vi "Post-Build Custom Action.vi"(10 "Variant":variant) -> (0 "error out":errorcluster)   [LabVIEW 2019]
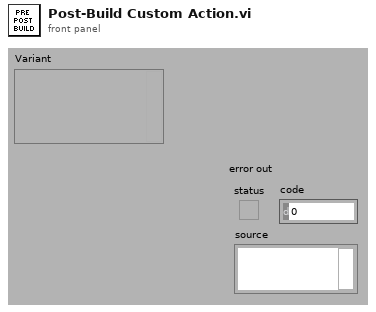
[diagram p1: front panel]
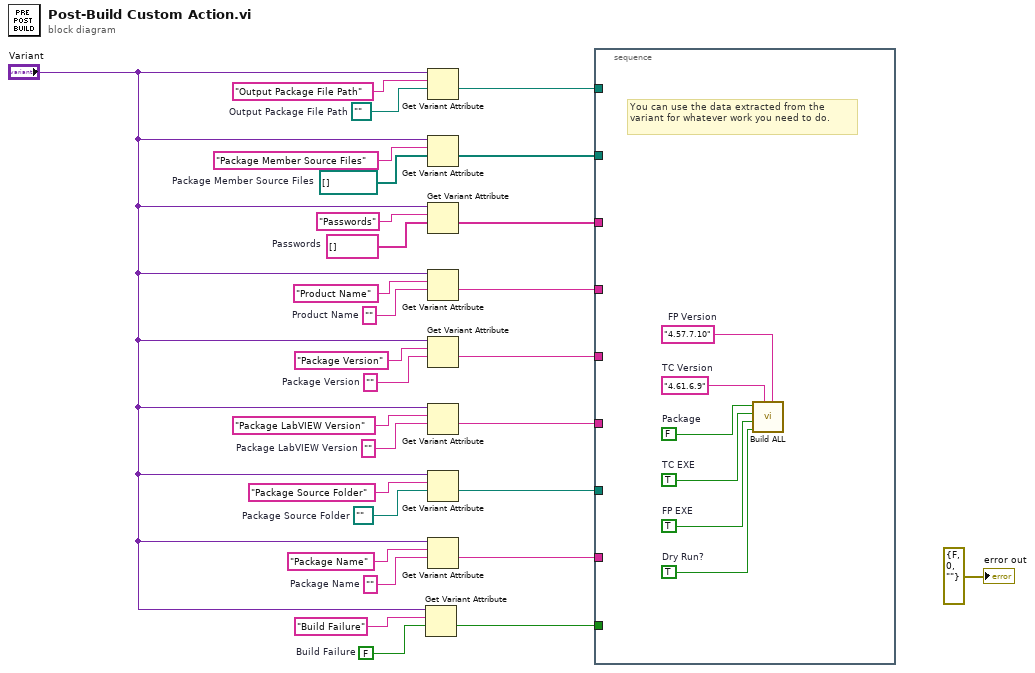
[diagram p0: block diagram]
diagram:
  w3 = FALSE  # Build Failure
  w13 = path ""  # Package Source Folder
  w14 = ""  # Package Name
  w17 = ""  # Package LabVIEW Version
  w19 = ""  # Package Version
  w21 = ""  # Product Name
  w24 = string[] []  # Passwords
  w26 = path[] []  # Package Member Source Files
  w28 = path ""  # Output Package File Path
  n1 = Get Variant Attribute(Variant="Variant", name="Build Failure", default value (empty Variant)=w3) -> (value=w1:bool)  [unwired: 1 in, 3 out]
  n2 = Get Variant Attribute(Variant="Variant", name="Output Package File Path", default value (empty Variant)=w28) -> (value=w12:path)  [unwired: 1 in, 3 out]
  n3 = Get Variant Attribute(Variant="Variant", name="Package Member Source Files", default value (empty Variant)=w26) -> (value=w11:path[])  [unwired: 1 in, 3 out]
  n4 = Get Variant Attribute(Variant="Variant", name="Passwords", default value (empty Variant)=w24) -> (value=w10:string[])  [unwired: 1 in, 3 out]
  n5 = Get Variant Attribute(Variant="Variant", name="Product Name", default value (empty Variant)=w21) -> (value=w9:string)  [unwired: 1 in, 3 out]
  n6 = Get Variant Attribute(Variant="Variant", name="Package Version", default value (empty Variant)=w19) -> (value=w8:string)  [unwired: 1 in, 3 out]
  n7 = Get Variant Attribute(Variant="Variant", name="Package LabVIEW Version", default value (empty Variant)=w17) -> (value=w7:string)  [unwired: 1 in, 3 out]
  n8 = Get Variant Attribute(Variant="Variant", name="Package Source Folder", default value (empty Variant)=w13) -> (value=w6:path)  [unwired: 1 in, 3 out]
  n9 = Get Variant Attribute(Variant="Variant", name="Package Name", default value (empty Variant)=w14) -> (value=w5:string)  [unwired: 1 in, 3 out]
  n10 = stacked-sequence {
    tunnel: w12 -> [_]
    tunnel: w11 -> [_]
    tunnel: w10 -> [_]
    tunnel: w9 -> [_]
    tunnel: w8 -> [_]
    tunnel: w7 -> [_]
    tunnel: w6 -> [_]
    tunnel: w5 -> [_]
    tunnel: w1 -> [_]
    frame #0 {
      w30 = FALSE  # Package
      w31 = TRUE  # TC EXE
      w32 = TRUE  # FP EXE
      w33 = TRUE  # Dry Run?
      w34 = "4.61.6.9"  # TC Version
      w35 = "4.57.7.10"  # FP Version
      # "You can use the data extracted from the variant for whatever work you need to do."
      n11 = call "Build ALL.vi"("FP Version"=w35, "TC Version"=w34, "Dry Run?"=w33, "FP EXE"=w32, "TC EXE"=w31, "Package"=w30) -> ()  [unwired: 6 in]
    }
  }
  "error out" <- errorcluster {"status"=FALSE, "code"=0, "source"=""} ("error out")
